vi "Standardize Multiple Angles in Radians.vi"(3 "angles in (rad)":dbl[](array[numeric]), 4 "range (-pi to pi)":T1=enum."-pi to pi") -> (5 "angles out (rad)":dbl[](array[numeric]))   [LabVIEW 2017, in "NI_Robotics Utilities.lvlib"]
doc: "Wraps a 1D array of angles in radians to be within a specific range.\n\nThis VI is deprecated. Use <vi.lib>\\Analysis\\coordinate.llb\\Wrap Angle.vi instead."
uses:
  <vilib>/robotics/Utilities/NI_Robotics Utilities.lvlib
  <vilib>/robotics/Utilities/Angle Range_Radians.ctl
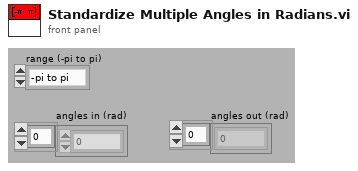
[diagram p1: front panel]
types:
  T1 = typedef "NI_Robotics Utilities.lvlib/Angle Range_Radians.ctl" = enum16{"none", "-pi to pi", "0 to 2*pi"}
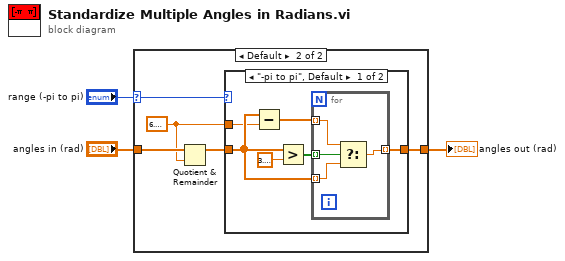
[diagram p0: block diagram]
diagram:
  n1 = case shown="Default" "range (-pi to pi)" {
    selector: "range (-pi to pi)" -> [_ w5]
    tunnel: "angles in (rad)" -> [w4 w9]
    tunnel: [w4 w8] -> w2
    frame "none" {
    }
    frame Default {
      w6 = 6.283185307179586
      n2 = Quotient & Remainder(x=w9, y=w6) -> (x-y*floor(x/y)=w7:dbl[])  [unwired: 1 out]
      n3 = case shown="\"-pi to pi\", Default" w5 {
        tunnel: [w14 w20] -> w8
        tunnel: w7 -> [w12 w20]
        tunnel: w6 -> [w11 _]
        frame "-pi to pi", Default {
          n4 = Subtract(x=w12, y=w11) -> (x-y=w10:dbl[])
          n5 = Greater?(x=w12, y=3.141592653589793) -> (0:w13:bool[])
          n6 = for {
            tunnel: w12 -> [w17] mode=indexing
            tunnel: w10 -> [w18] mode=indexing
            tunnel: [w16] -> w14 mode=indexing
            tunnel: w13 -> [w19] mode=indexing
            n7 = Select(t=w18, s=w19, f=w17) -> (s? t:f=w16:dbl)
          }
        }
        frame "0 to 2*pi" {
        }
      }
    }
  }
  "angles out (rad)" <- w2
